vi "Example.vi"() -> ()   [LabVIEW 2018]
uses:
  Data Def/IT8800-Operation Mode.ctl
  Data Def/IT8800-Setting.ctl
  VI/IT8800-Configure Constant Voltage.vi
  VI/IT8800-Configure Constant Power.vi
  VI/IT8800-Configure Constant Resistance.vi
  VI/IT8800-Configure Constant Current.vi
panel:
  out "loop time":u32
  in  "Numeric":dbl format="%#_13g"
  in  "Range Type":T1
  in  "Apply Range":bool
  out "Operation Mode":T1
  out "Limits":dbl[][](array[numeric])
  out "error IO":errorcluster
  out "Elapsed Time (Sec)":dbl
  in  "Apply":bool
  in  "Value":dbl=5.0
  in  "Operation Mode":T1
  out "Input?":bool
  in  "Stop Load":bool
  in  "Apply Load":bool
  out "Chart":T2(graph)={"Voltage (Volts)"=-1.0, "Power (Watts)"=-1.0, "Current (Amps)"=-1.0}
  out "Stop?":bool
  in  "IT8800 Setting In In":T3={"VISA Resource Name"="COM4", "Baud Rate"=9600, "Stop Bits"=10, "Wait For Read(ms)"=10} {"Stop Bits" items=["1.0"=10, "2.0"=20]; "Baud Rate" items=["2400"=2400, "4800"=4800, "9600"=9600, "19200"=19200]}
  # "Current"
  # "Voltage"
  # "Power"
  # "Ressitance"
  # "uplimit"
  # "downlimit"
  # "range"
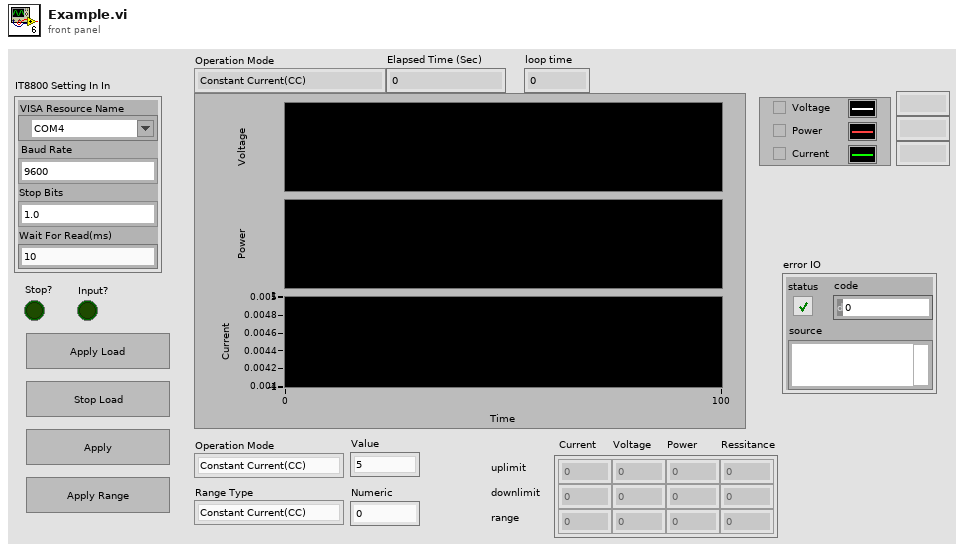
[diagram p1: front panel]
types:
  T1 = typedef "IT8800-Operation Mode.ctl" = enum16{"Constant Current(CC)", "Constant Voltage(CV)", "Constant Power(CP)", "Constant Resistance(CR)"}
  T2 = cluster{"Voltage (Volts)":dbl, "Power (Watts)":dbl, "Current (Amps)":dbl}
  T3 = cluster{"VISA Resource Name":refnum<visa-resource-name>, "Baud Rate":u32, "Stop Bits":u16, "Wait For Read(ms)":u32}
  T4 = typedef "IT8800-Setting.ctl" = cluster{"VISA Resource Name":refnum<visa-resource-name>, "Baud Rate":u32, "Stop Bits":u16, "Wait For Read(ms)":u32, "Interface Type":enum16{"Unknow", "GPIB", "VXI", "GPIB-VXI", "Serial", "PXI", "TCPIP", "USB", "FireWire"}, "Limits":dbl[][]}
  T5 = typedef "IT8800-Measurement Data.ctl" = cluster{"Current (Amps)":dbl, "Power (Watts)":dbl, "Voltage (Volts)":dbl, "Elapsed Time (Sec) ":dbl}
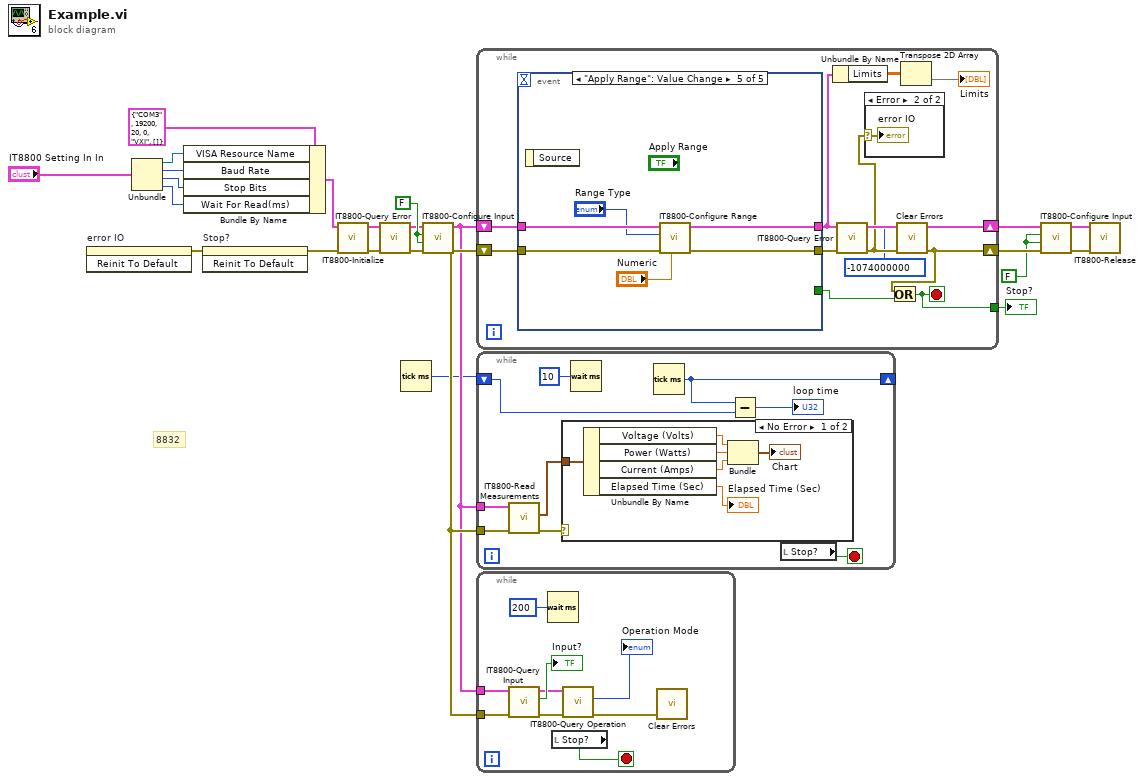
[diagram p0: block diagram]
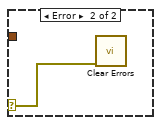
[diagram p2: hidden frame]
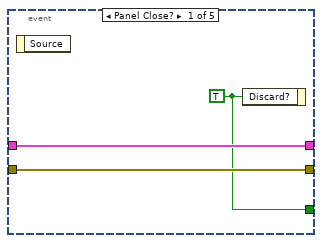
[diagram p4: hidden frame]
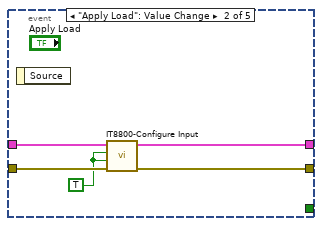
[diagram p5: hidden frame]
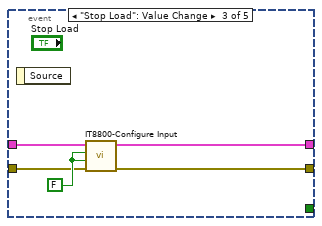
[diagram p6: hidden frame]
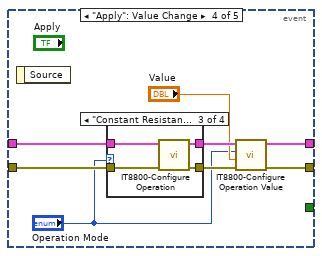
[diagram p7: hidden frame]
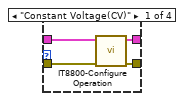
[diagram p8: hidden frame]
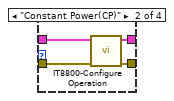
[diagram p9: hidden frame]
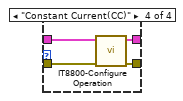
[diagram p10: hidden frame]
diagram:
  w18 = FALSE ("Enable Input")
  w23 = FALSE ("Enable Input")
  # "8832"
  n1 = invoke on="error IO" class="Clust (strict)" method="Reinit To Default"() -> (error out=w3:errorcluster)  [unwired: 3 in, 2 out]
  n2 = Unbundle("IT8800 Setting In In") -> ("VISA Resource Name"=w8:refnum<visa-resource-name>, "Baud Rate"=w7:u32, "Stop Bits"=w6:u16, "Wait For Read(ms)"=w5:u32)
  n3 = Bundle By Name(cluster=T4 {"VISA Resource Name"="COM3", "Baud Rate"=19200, "Stop Bits"=20, "Wait For Read(ms)"=0, "Interface Type"=enum."VXI", "Limits"=[]} ("ITech Setting In"), "VISA Resource Name"=w8, "Baud Rate"=w7, "Stop Bits"=w6, "Wait For Read(ms)"=w5) -> (w4:T4)
  n4 = invoke on="Stop?" class="Bool (strict)" method="Reinit To Default"(error in=w3) -> (error out=w17:errorcluster)  [unwired: 2 in, 2 out]
  n5 = call "IT8800-Initialize.vi"("error in (no error)"=w17, "ITech Setting In"=w4) -> ("error out"=w13:errorcluster, "IT8800 Setting In Out"=w15:T4)  [unwired: 8 in]
  n6 = call "IT8800-Query Error.vi"("error in"=w13, "IT8800 Setting In In"=w15) -> ("error out"=w12:errorcluster, "IT8800 Setting In Out"=w14:T4)  [unwired: 8 in]
  n7 = Tick Count (ms)() -> (millisecond timer value=w1:u32)
  n8 = call "IT8800-Configure Input.vi"("error in"=w12, "Enable Input Short"=w23, "Enable Input"=w23, "IT8800 Setting In In"=w14) -> ("error out"=w11:errorcluster, "IT8800 Setting In Out"=w2:T4)  [unwired: 6 in]
  n9 = while {
    tunnel: [w28] -> w16
    shift-right: [w32] -> w22
    shift-left: w2 -> [w34]
    shift-right: [w27] -> w21
    shift-left: w11 -> [w35]
    stop <- w28 stop-if-true
    n10 = event shown="[4] \"Apply Range\": Value Change" {
      selector: _ -> [_ _ _ _ _]
      dyn-events: _ -> [_ _ _ _ _]
      timeout: _ -> [_ _ _ _ _]
      tunnel: w35 -> [w39 w43 w47 w51 w78]
      tunnel: w34 -> [w38 w44 w48 w52 w79]
      tunnel: [w39 w41 w45 w54 w76] -> w31
      tunnel: [w37 _ _ _ _] -> w33
      tunnel: [w38 w42 w46 w55 w77] -> w24
      event Panel Close? {
        w37 = TRUE ("Discard?")
        n11 = event-data() -> ()  [unwired: 1 in, 1 out]
        n12 = event-data("Discard?"=w37) -> ()  [unwired: 1 in, 1 out]
      }
      event "Apply Load": Value Change {
        w40 = TRUE ("Enable Input")
        n13 = event-data() -> ()  [unwired: 1 in, 1 out]
        n14 = call "IT8800-Configure Input.vi"("error in"=w43, "Enable Input Short"=w40, "Enable Input"=w40, "IT8800 Setting In In"=w44) -> ("error out"=w41:errorcluster, "IT8800 Setting In Out"=w42:T4)  [unwired: 6 in]
      }
      event "Stop Load": Value Change {
        w49 = FALSE ("Enable Input")
        n15 = event-data() -> ()  [unwired: 1 in, 1 out]
        n16 = call "IT8800-Configure Input.vi"("error in"=w47, "Enable Input Short"=w49, "Enable Input"=w49, "IT8800 Setting In In"=w48) -> ("error out"=w45:errorcluster, "IT8800 Setting In Out"=w46:T4)  [unwired: 6 in]
      }
      event "Apply": Value Change {
        n17 = event-data() -> ()  [unwired: 1 in, 1 out]
        n18 = case shown="\"Constant Resistance(CR)\"" "Operation Mode" {
          tunnel: [w61 w65 w69 w73] -> w57
          tunnel: [w60 w64 w68 w72] -> w56
          tunnel: w52 -> [w59 w63 w67 w71]
          tunnel: w51 -> [w58 w62 w66 w70]
          frame "Constant Voltage(CV)" {
            n19 = call-poly "IT8800-Configure Operation.vi"("error in"=w58, "IT8800 Setting In In"=w59) -> ("error out"=w60:errorcluster, "IT8800 Setting In Out"=w61:T4)  [unwired: 8 in]
          }
          frame "Constant Power(CP)" {
            n20 = call-poly "IT8800-Configure Operation.vi"("error in"=w62, "IT8800 Setting In In"=w63) -> ("error out"=w64:errorcluster, "IT8800 Setting In Out"=w65:T4)  [unwired: 8 in]
          }
          frame "Constant Resistance(CR)" {
            n21 = call-poly "IT8800-Configure Operation.vi"("error in"=w66, "IT8800 Setting In In"=w67) -> ("error out"=w68:errorcluster, "IT8800 Setting In Out"=w69:T4)  [unwired: 8 in]
          }
          frame "Constant Current(CC)" {
            n22 = call-poly "IT8800-Configure Operation.vi"("error in"=w70, "IT8800 Setting In In"=w71) -> ("error out"=w72:errorcluster, "IT8800 Setting In Out"=w73:T4)  [unwired: 8 in]
          }
        }
        n23 = call "IT8800-Configure Operation Value.vi"("error in"=w56, "Values (0)"="Value", "Value Type (0:Current)"="Operation Mode", "IT8800 Setting In In"=w57) -> ("error out"=w54:errorcluster, "IT8800 Setting In Out"=w55:T4)  [unwired: 6 in]
      }
      event "Apply Range": Value Change {
        n24 = event-data() -> ()  [unwired: 1 in, 1 out]
        n25 = call "IT8800-Configure Range.vi"("Numeric"="Numeric", "error in"=w78, "Range Type"="Range Type", "IT8800 Setting In In"=w79) -> ("error out"=w76:errorcluster, "IT8800 Setting In Out"=w77:T4)  [unwired: 6 in]
      }
    }
    n26 = Unbundle By Name(w24) -> ("Limits"=w25:dbl[][])
    n27 = call "IT8800-Query Error.vi"("error in"=w31, "IT8800 Setting In In"=w24) -> ("error out"=w30:errorcluster, "IT8800 Setting In Out"=w32:T4)  [unwired: 8 in]
    n28 = case shown="Error" w30 {
      selector: w30 -> [_ w36]
      frame No Error {
      }
      frame Error {
        "error IO" <- w36
      }
    }
    n29 = call <vilib>:"Clear Errors.vi"("error in (no error)"=w30, "specific error code to clear (0: all)"=-1074000000) -> ("error out"=w27:errorcluster)  [unwired: 4 in, 1 out]
    n30 = Or(x=w27, y=w33) -> (x .or. y?=w28:bool)
    n31 = Transpose 2D Array(2D array=w25) -> (transposed array=→"Limits":dbl[][])
  }
  "Stop?" <- w16
  n32 = while {
    tunnel: w2 -> [w86]
    tunnel: w11 -> [w87]
    shift-right: [w83] -> _
    shift-left: w1 -> [w82]
    stop <- w88 stop-if-true
    n33 = call "IT8800-Read Measurements.vi"("error in"=w87, "IT8800 Setting In In"=w86) -> ("error out"=w84:errorcluster, "Measurement Data"=w85:T5)  [unwired: 7 in, 1 out]
    n34 = case shown="No Error" w84 {
      selector: w84 -> [_ w95]
      tunnel: w85 -> [w94 _]
      frame No Error {
        n35 = Unbundle By Name(w94) -> ("Voltage (Volts)"=w93:dbl, "Power (Watts)"=w92:dbl, "Current (Amps)"=w91:dbl, "Elapsed Time (Sec)"=→"Elapsed Time (Sec)":dbl)
        n36 = Bundle("Voltage (Volts)"=w93, "Power (Watts)"=w92, "Current (Amps)"=w91) -> (→"Chart":T2)  [unwired: 1 in]
      }
      frame Error {
        n37 = call <vilib>:"Clear Errors.vi"("error in (no error)"=w95) -> ()  [unwired: 5 in, 2 out]
      }
    }
    n38 = Wait (ms)(milliseconds to wait=u32 10) -> ()  [unwired: 1 out]
    n39 = Tick Count (ms)() -> (millisecond timer value=w83:u32)
    n40 = Subtract(x=w83, y=w82) -> (x-y=→"loop time":u32)
    n41 = local read "Stop?"() -> (w88:bool)
  }
  n42 = while {
    tunnel: w2 -> [w101]
    tunnel: w11 -> [w102]
    stop <- w104 stop-if-true
    n43 = call "IT8800-Query Input.vi"("error in"=w102, "IT8800 Setting In In"=w101) -> ("error out"=w97:errorcluster, "Input?"=→"Input?":bool, "IT8800 Setting In Out"=w98:T4)  [unwired: 7 in]
    n44 = Wait (ms)(milliseconds to wait=u32 200) -> ()  [unwired: 1 out]
    n45 = local read "Stop?"() -> (w104:bool)
    n46 = call "IT8800-Query Operation.vi"("error in"=w97, "IT8800 Setting In In"=w98) -> ("error out"=w96:errorcluster, "Operation Mode"=→"Operation Mode":T1)  [unwired: 7 in, 1 out]
    n47 = call <vilib>:"Clear Errors.vi"("error in (no error)"=w96) -> ()  [unwired: 5 in, 2 out]
  }
  n48 = call "IT8800-Configure Input.vi"("error in"=w21, "Enable Input Short"=w18, "Enable Input"=w18, "IT8800 Setting In In"=w22) -> ("error out"=w19:errorcluster, "IT8800 Setting In Out"=w20:T4)  [unwired: 6 in]
  n49 = call "IT8800-Release.vi"("error in"=w19, "IT8800 Setting In"=w20) -> ()  [unwired: 9 in, 1 out]
